vi "Traffic_Control.vi"() -> ()   [LabVIEW 2020]
panel:
  out "Green":bool
  out "Yellow":bool
  out "Red":bool
  # "Traffic Signals"
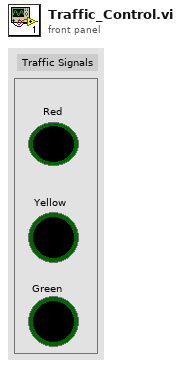
[diagram p1: front panel]
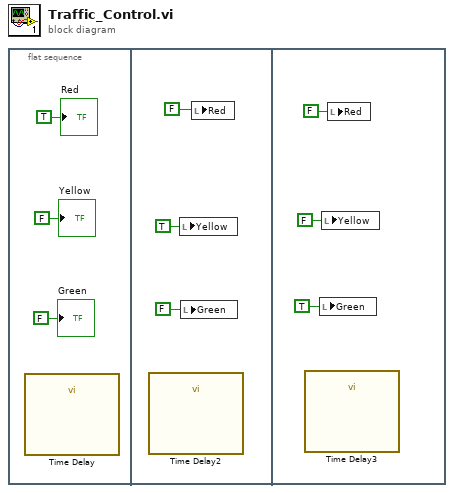
[diagram p0: block diagram]
diagram:
  n1 = flat-sequence {
    frame #0 {
      n2 = call "Time Delay"() -> ()  [unwired: 11 in, 1 out]
      "Red" <- TRUE ("Red")
      "Yellow" <- FALSE ("Yellow")
      "Green" <- FALSE ("Greean")
    }
    frame #1 {
      n3 = call "Time Delay2"() -> ()  [unwired: 11 in, 1 out]
      n4 = local write "Yellow"(TRUE ("Yellow")) -> ()
      n5 = local write "Green"(FALSE ("Greean")) -> ()
      n6 = local write "Red"(FALSE ("Red")) -> ()
    }
    frame #2 {
      n7 = call "Time Delay3"() -> ()  [unwired: 11 in, 1 out]
      n8 = local write "Green"(TRUE ("Greean")) -> ()
      n9 = local write "Yellow"(FALSE ("Yellow")) -> ()
      n10 = local write "Red"(FALSE ("Red")) -> ()
    }
  }
